vi "Interface_Asset_Write Asset.vi"(8 "error in (no error)":errorcluster, 10 "TagBus DVR":refnum<data-value>, 11 "Asset_Interface in":refnum<class "Interface_Asset.lvclass">) -> (0 "error out":errorcluster, 2 "TagBus DVR out":refnum<data-value>, 3 "Asset_Interface out":refnum<class "Interface_Asset.lvclass">)   [LabVIEW 2015, in "Interface_Asset.lvclass"]
uses:
  Interface_Asset.lvclass
  TagBus/TagBus.lvclass
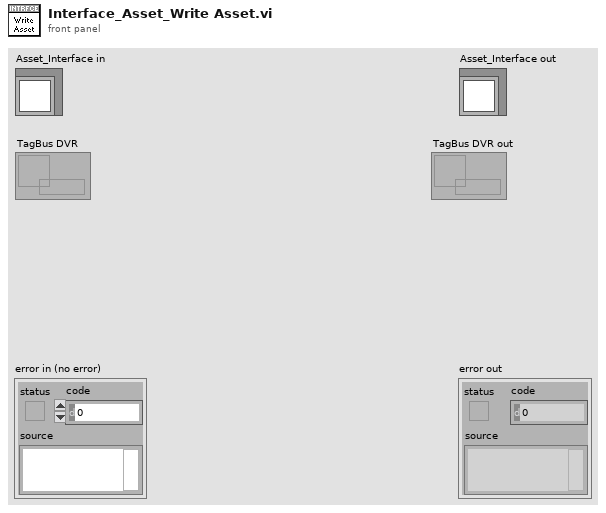
[diagram p1: front panel]
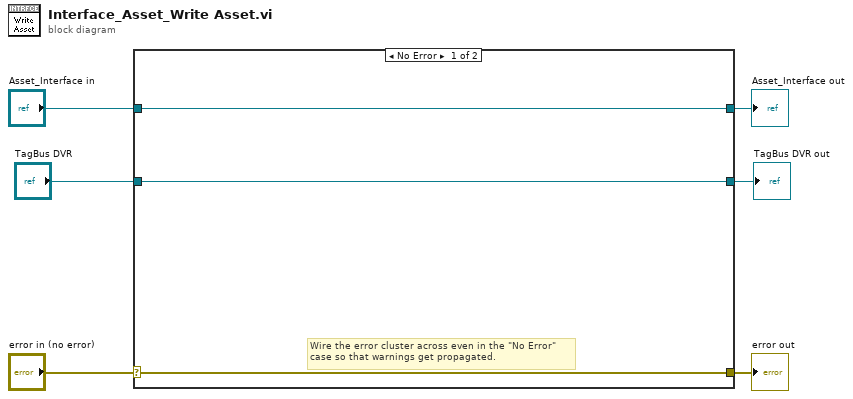
[diagram p0: block diagram]
diagram:
  n1 = case shown="No Error" "error in (no error)" {
    selector: "error in (no error)" -> [w8 w12]
    tunnel: [w8 w12] -> w5
    tunnel: [w9 w11] -> w3
    tunnel: "Asset_Interface in" -> [w9 w11]
    tunnel: [w7 w10] -> w2
    tunnel: "TagBus DVR" -> [w7 w10]
    frame No Error {
      # "Wire the error cluster across even in the \"No Error\"\ncase so that warnings get propagated."
    }
    frame Error {
    }
  }
  "error out" <- w5
  "Asset_Interface out" <- w3
  "TagBus DVR out" <- w2
